vi "GetExportModel.vi"(6 "型号":u16(ring) caption="产品型号" items=["90-18", "90-88"], 7 "产品种类":u16(ring) items=["外购带卡", "外购不带卡", "自产"], 8 "error in":errorcluster caption="错误输入", 9 "型号":refnum<vi>, 10 "Debug":bool, 11 "产品类型":refnum<vi>) -> (0 "error out":errorcluster caption="错误输出")   [LabVIEW 2013]
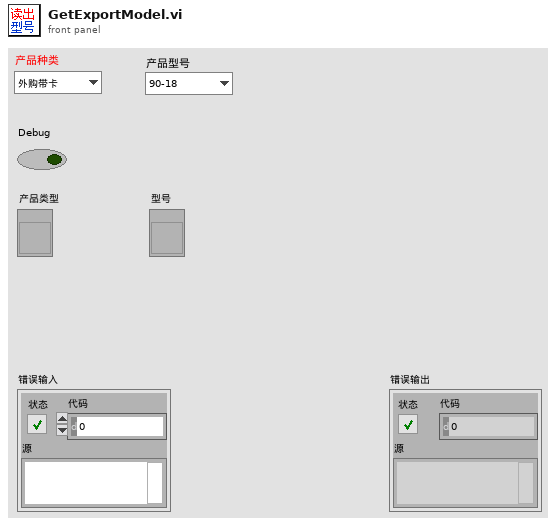
[diagram p1: front panel]
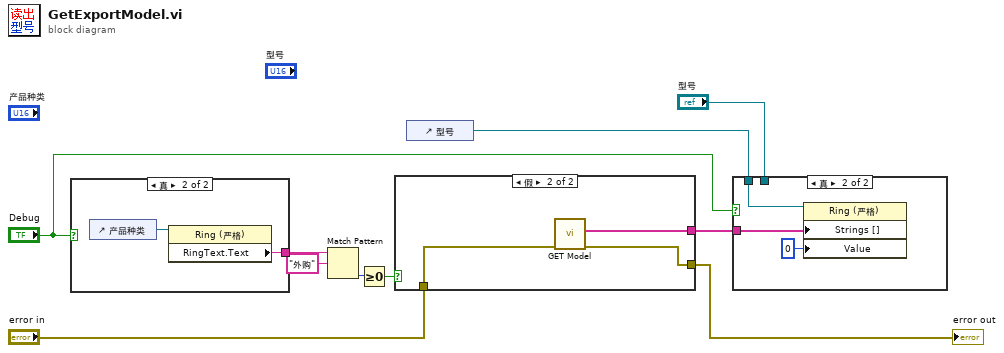
[diagram p0: block diagram]
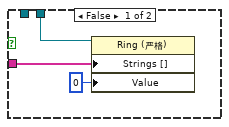
[diagram p2: hidden frame]
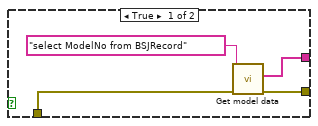
[diagram p3: hidden frame]
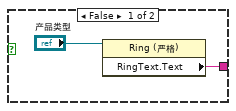
[diagram p4: hidden frame]
diagram:
  n1 = case shown="真" "Debug" {
    tunnel: [w11 w14] -> w4
    frame False {
      n2 = property class="Ring (严格)"(reference="产品类型") -> ("RingText.Text"=w11:string)  [unwired: 1 in, 2 out]
    }
    frame True {
      n3 = control-ref of="产品种类"() -> (w13:refnum<vi>)
      n4 = property class="Ring (严格)"(reference=w13) -> ("RingText.Text"=w14:string)  [unwired: 1 in, 2 out]
    }
  }
  n5 = Match Pattern(string=w4, regular expression="外购" ("正则表达式")) -> (offset past match=w2:i32)  [unwired: 1 in, 3 out]
  n6 = Greater Or Equal To 0?(x=w2) -> (x >= 0?=w1:bool)
  n7 = case shown="假" w1 {
    tunnel: [w17 w21] -> w5
    tunnel: "error in" -> [w16 w20]
    tunnel: [w15 w19] -> w9
    frame True {
      n8 = call "Get model data.vi"("error in (no error)"=w16, "CMD_Str"="select ModelNo from BSJRecord") -> ("error out"=w15:errorcluster, "Model Names"=w17:string[])  [unwired: 8 in]
    }
    frame False {
      n9 = call "GET Model.vi"("error in"=w20) -> ("error out"=w19:errorcluster, "Model Names"=w21:string[])  [unwired: 9 in]
    }
  }
  "error out" <- w9
  n10 = control-ref of="型号"() -> (w7:refnum<vi>)
  n11 = case shown="真" "Debug" {
    tunnel: w7 -> [_ w26]
    tunnel: "型号" -> [w23 _]
    tunnel: w5 -> [w22 w25]
    frame False {
      n12 = property class="Ring (严格)"(reference=w23, "Strings []"=w22, "Value"=u16 0 ("值")) -> ()  [unwired: 1 in, 2 out]
    }
    frame True {
      n13 = property class="Ring (严格)"(reference=w26, "Strings []"=w25, "Value"=u16 0 ("值")) -> ()  [unwired: 1 in, 2 out]
    }
  }
